vi "DAQ-Hybrid Engine-final.vi"() -> ()   [LabVIEW 2013]
uses:
  <vilib>/DAQmx/read.llb/DAQmx Read (Analog 1D Wfm NChan 1Samp).vi
  <vilib>/Analysis/baseanly.llb/Mean (DBL).vi
  <vilib>/DAQmx/read.llb/DAQmx Read (Analog Wfm 1Chan NSamp).vi
  <vilib>/DAQmx/read.llb/DAQmx Read (Analog Wfm 1Chan 1Samp).vi
  <vilib>/DAQmx/read.llb/DAQmx Read (Analog 1D DBL NChan 1Samp).vi
  <vilib>/DAQmx/configure/timing.llb/DAQmx Timing (Sample Clock).vi
  <vilib>/Utility/file.llb/Write To Spreadsheet File (string).vi
  <vilib>/Utility/file.llb/Write To Spreadsheet File (DBL).vi
  <vilib>/DAQmx/miscellaneous.llb/DAQmx Fill In Error Info.vi
  <vilib>/Analysis/NI_AALBase.lvlib
panel:
  in  "clear chart":bool
  out "?":dbl
  out "Servo":dbl(slide)=-430.10425378048984 scale=0.0..100.0
  out "?":dbl
  out "Chamber":dbl(slide)=-430.2760122999443 scale=0.0..100.0
  out "?":dbl
  out "Plumbing":dbl(slide)=-430.905793537944 scale=0.0..100.0
  out "?":dbl
  out "Pressure 2":dbl(knob) scale=0.0..2000.0
  in  "File Path 3":path=path "C:/Users/local-admin/Desktop/SRT-3 DAQ/test117.csv"
  out "?":dbl
  out "Ambient":dbl(slide)=-430.10425378048984 scale=0.0..100.0
  out "Waveform Chart":waveform(dbl)(graph)={"t0"=timestamp(3542319786.47639 s since 1904-01-01), "dt"=0.1, "Y"=[-147.1278504434858, -147.1152908145616], "attributes"=variant("NI_ChannelName"=variant(string "Voltage"), "NI_UnitDescription"=variant(string "Lbf"))}
  out "?":dbl
  out "Thrust":dbl(slide)=1.707317073170724 scale=-350.0..350.0
  out "?":dbl
  out "Plumbing":dbl(knob) scale=0.0..2000.0
  in  "?":bool
  in  "Samples Per Update":dbl=10.0
  in  "Sampling Rate [Hz]":i32=10
  # "Sampling Settings"
  # "Data Logging Settings"
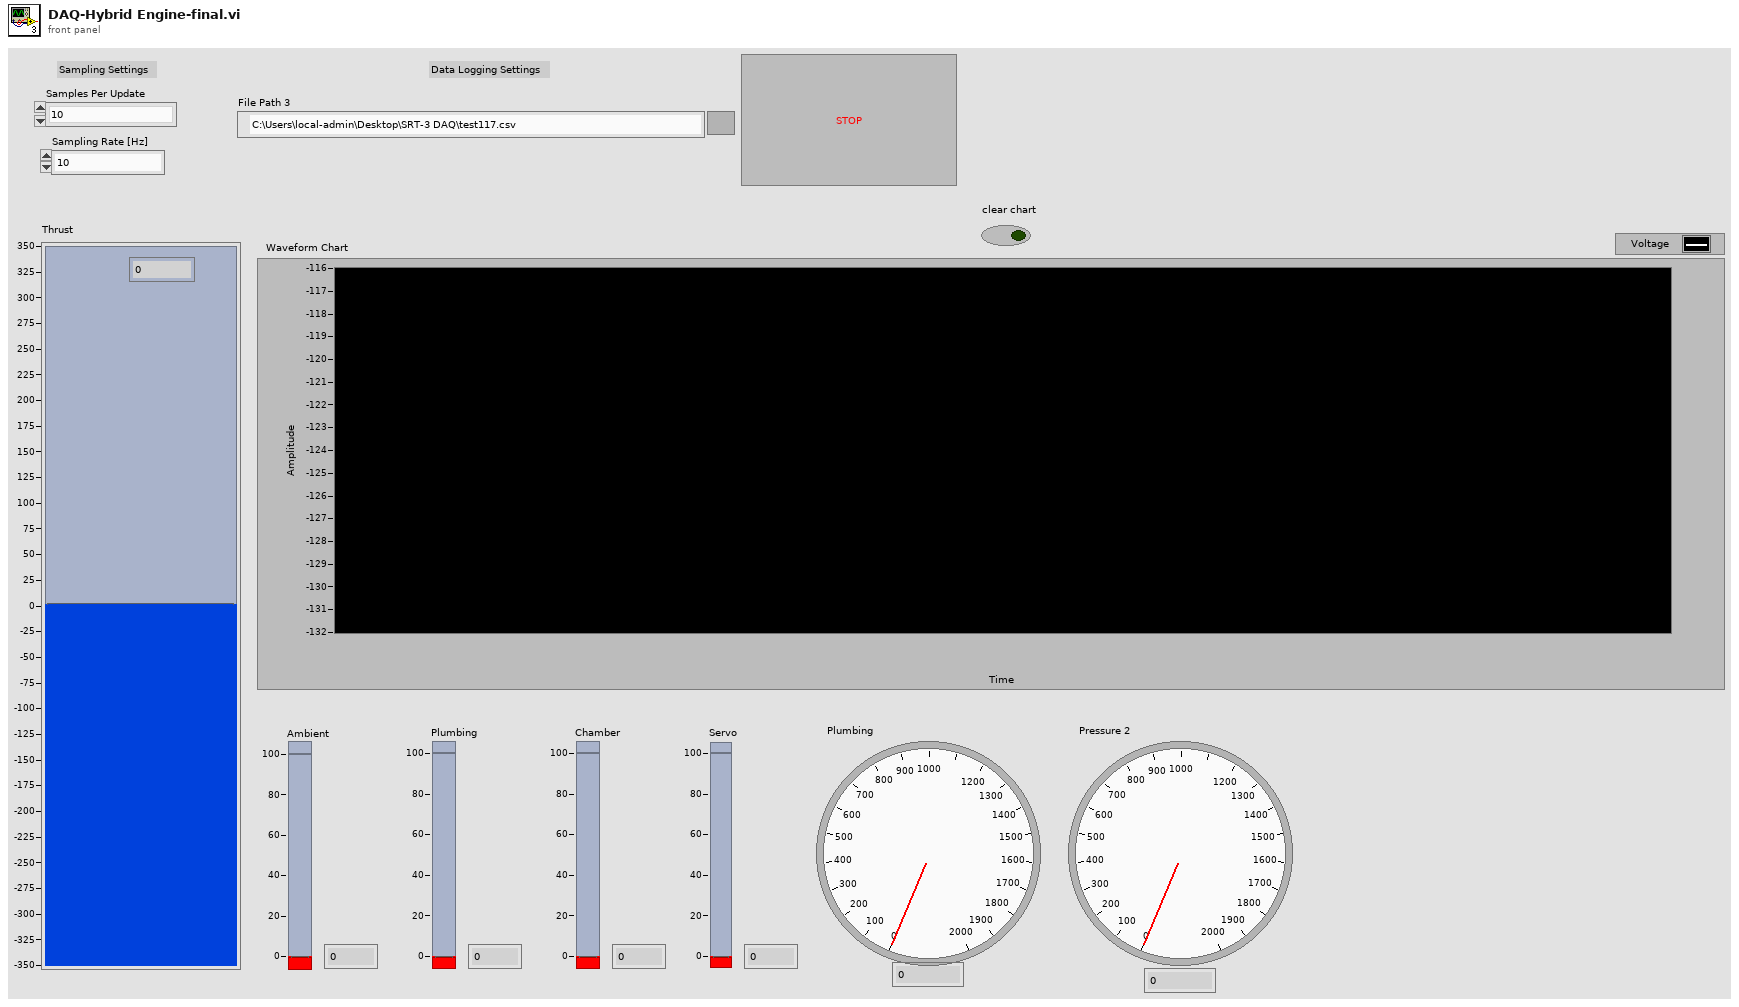
[diagram p1: front panel]
types:
  T1 = enum16{"open", "replace", "create", "open or create", "replace or create", "replace or create with confirmation"}
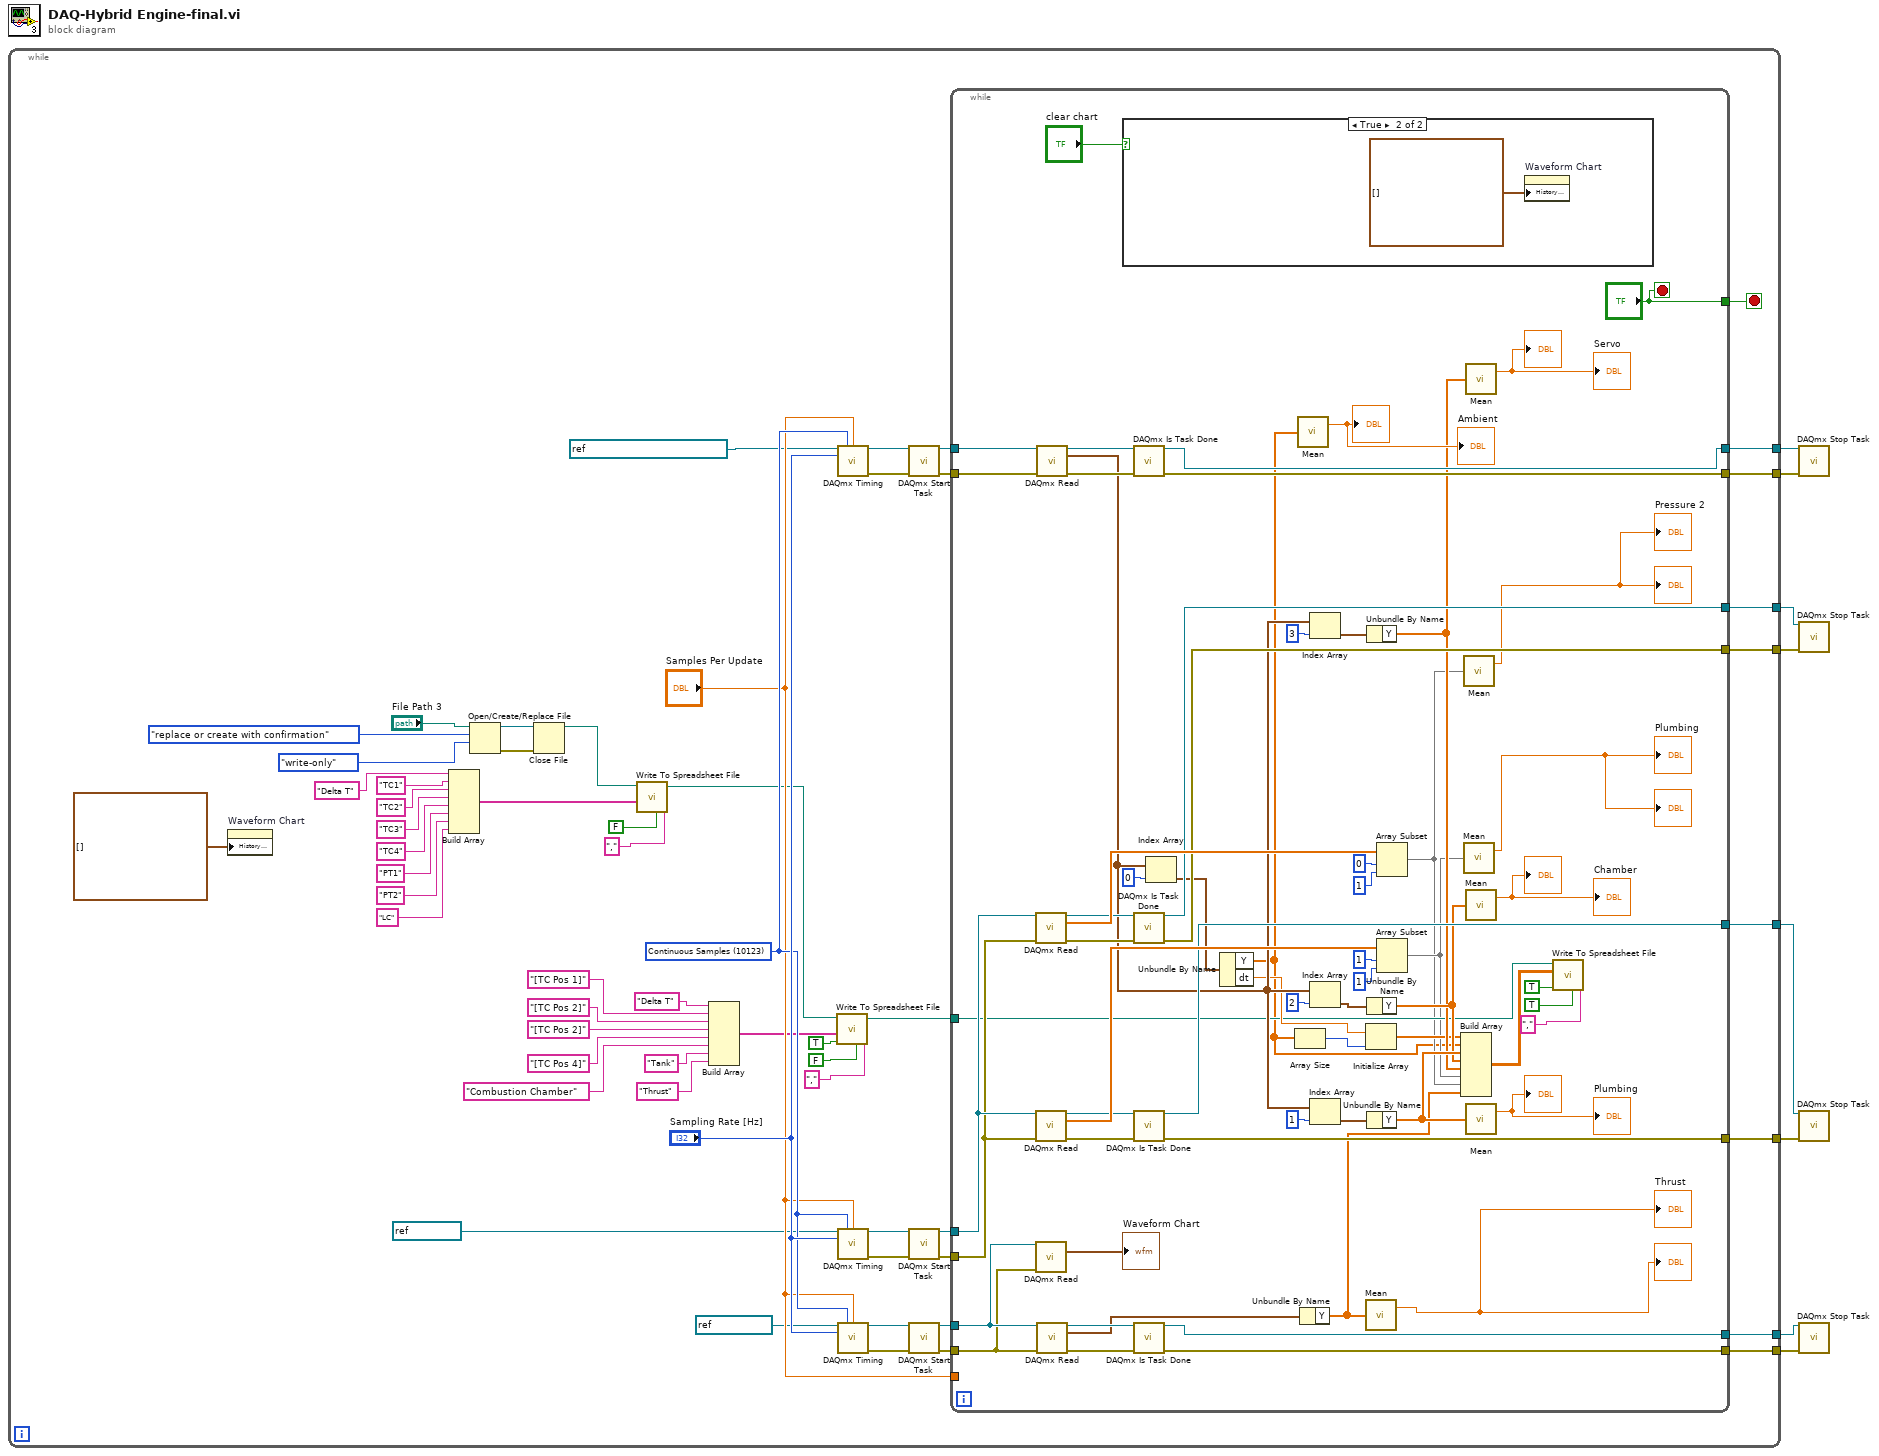
[diagram p0: block diagram]
diagram:
  n1 = while {
    tunnel: [w54] -> w8
    tunnel: [w53] -> w7
    tunnel: [w56] -> w6
    tunnel: [w55] -> w5
    tunnel: [w52] -> w4
    tunnel: [w51] -> w3
    tunnel: [w50] -> w2
    tunnel: [w49] -> w1
    stop <- w11 stop-if-true
    w61 = 10123 items=["Finite Samples"=10178, "Continuous Samples"=10123, "Hardware Timed Single Point"=12522] ("sample mode")
    n2 = property on="Waveform Chart" class="WFChart (strict)"("History Data"=waveform(dbl)[] []) -> ()  [unwired: 2 in, 2 out]
    n3 = Build Array("Delta T", "TC1", "TC2", "TC3", "TC4", "PT1", "PT2", "LC") -> (w31:string[])
    n4 = Open/Create/Replace File(file path (use dialog)="File Path 3", operation (0:open)=T1."replace or create with confirmation", access (0:read/write)=enum16{"read/write", "read-only", "write-only"}."write-only") -> (refnum out=w45:refnum<file>, error out=w44:errorcluster)  [unwired: 3 in, 1 out]
    n5 = Close File(refnum=w45, error in=w44) -> (path=w34:path)  [unwired: 1 out]
    n6 = call-poly <vilib>:"Write To Spreadsheet File.vi"("delimiter (\\t)"="," ("delimiter (\\t)"), "transpose? (no:F)"=FALSE, "1D data"=w31, "file path (dialog if empty)"=w34) -> ("new file path (Not A Path if cancelled)"=w20:path)  [unwired: 4 in]
    n7 = Build Array("Delta T", "[TC Pos 1]", "[TC Pos 2]", "[TC Pos 2]", "[TC Pos 4]", "Combustion Chamber", "Tank", "Thrust") -> (w16:string[])
    n8 = call-poly <vilib>:"Write To Spreadsheet File.vi"("delimiter (\\t)"="," ("delimiter (\\t)"), "transpose? (no:F)"=FALSE, "append to file? (new file:F)"=TRUE, "1D data"=w16, "file path (dialog if empty)"=w20) -> ("new file path (Not A Path if cancelled)"=w14:path)  [unwired: 3 in]
    n9 = call-poly <vilib>:"DAQmx Timing.vi"("task/channels in"=refnum<k21> "Thermocouple Channels" ("task in"), "sample mode"=w61, "samples per channel"="Samples Per Update", "rate"="Sampling Rate [Hz]") -> ("task out"=w59:refnum<k21>, "error out"=w58:errorcluster)  [unwired: 10 in]
    n10 = call-poly <vilib>:"DAQmx Timing.vi"("task/channels in"=refnum<k21> "PT 2000" ("task in"), "sample mode"=w61, "samples per channel"="Samples Per Update", "rate"="Sampling Rate [Hz]") -> ("task out"=w43:refnum<k21>, "error out"=w42:errorcluster)  [unwired: 10 in]
    n11 = call-poly <vilib>:"DAQmx Timing.vi"("task/channels in"=refnum<k21> "Load Cell" ("task in"), "sample mode"=w61, "samples per channel"="Samples Per Update", "rate"="Sampling Rate [Hz]") -> ("task out"=w41:refnum<k21>, "error out"=w40:errorcluster)  [unwired: 10 in]
    n12 = call <vilib>:"DAQmx Start Task.vi"("task/channels in"=w59, "error in"=w58) -> ("task out"=w63:refnum<k21>, "error out"=w57:errorcluster)  [unwired: 12 in]
    n13 = call <vilib>:"DAQmx Start Task.vi"("task/channels in"=w43, "error in"=w42) -> ("task out"=w67:refnum<k21>, "error out"=w66:errorcluster)  [unwired: 12 in]
    n14 = call <vilib>:"DAQmx Start Task.vi"("task/channels in"=w41, "error in"=w40) -> ("task out"=w65:refnum<k21>, "error out"=w64:errorcluster)  [unwired: 12 in]
    n15 = while {
      tunnel: w67 -> [w110]
      tunnel: w66 -> [w109]
      tunnel: ["?"] -> w11
      tunnel: w65 -> [w76]
      tunnel: w64 -> [w75]
      tunnel: "Samples Per Update" -> [_]
      tunnel: w63 -> [w101]
      tunnel: w57 -> [w127]
      tunnel: [w119] -> w56
      tunnel: [w118] -> w55
      tunnel: [w117] -> w54
      tunnel: [w116] -> w53
      tunnel: [w108] -> w52
      tunnel: [w107] -> w51
      tunnel: [w106] -> w50
      tunnel: [w105] -> w49
      tunnel: w14 -> [w81]
      stop <- "?" stop-if-true
      n16 = call-poly <vilib>:"DAQmx Read.vi"("task/channels in"=w110, "error in"=w109) -> ("task out"=w111:refnum<k21>, "data"=w114:dbl[], "error out"=w112:errorcluster)  [unwired: 11 in]
      n17 = call-poly <vilib>:"DAQmx Read.vi"("task/channels in"=w110, "error in"=w109) -> ("task out"=w124:refnum<k21>, "data"=w129:dbl[], "error out"=w125:errorcluster)  [unwired: 11 in]
      n18 = call-poly <vilib>:"DAQmx Read.vi"("task/channels in"=w76, "error in"=w75) -> ("data"=→"Waveform Chart":waveform(dbl))  [unwired: 11 in, 2 out]
      n19 = call-poly <vilib>:"DAQmx Read.vi"("task/channels in"=w101, "error in"=w127) -> ("task out"=w122:refnum<k21>, "data"=w97:waveform(dbl)[], "error out"=w123:errorcluster)  [unwired: 11 in]
      n20 = call-poly <vilib>:"DAQmx Read.vi"("task/channels in"=w76, "error in"=w75) -> ("task out"=w120:refnum<k21>, "data"=w74:waveform(dbl), "error out"=w121:errorcluster)  [unwired: 11 in]
      n21 = case shown="True" "clear chart" {
        frame False {
        }
        frame True {
          n22 = property on="Waveform Chart" class="WFChart (strict)"("History Data"=waveform(dbl)[] []) -> ()  [unwired: 2 in, 2 out]
        }
      }
      n23 = call <vilib>:"DAQmx Is Task Done.vi"("task/channels in"=w122, "error in"=w123) -> ("task out"=w106:refnum<k21>, "error out"=w105:errorcluster)  [unwired: 11 in, 1 out]
      n24 = call <vilib>:"DAQmx Is Task Done.vi"("task/channels in"=w111, "error in"=w112) -> ("task out"=w108:refnum<k21>, "error out"=w107:errorcluster)  [unwired: 11 in, 1 out]
      n25 = call <vilib>:"DAQmx Is Task Done.vi"("task/channels in"=w124, "error in"=w125) -> ("task out"=w117:refnum<k21>, "error out"=w116:errorcluster)  [unwired: 11 in, 1 out]
      n26 = call <vilib>:"DAQmx Is Task Done.vi"("task/channels in"=w120, "error in"=w121) -> ("task out"=w119:refnum<k21>, "error out"=w118:errorcluster)  [unwired: 11 in, 1 out]
      n27 = Index Array(array=w97, index=0) -> (element=w96:waveform(dbl))
      n28 = Unbundle By Name(w96) -> ("Y"=w78:dbl[], "dt"=w83:dbl)
      n29 = Array Size(array=w78) -> (size(s)=w84:i32)
      n30 = call-poly <vilib>:"Mean.vi"("X"=w78) -> ("mean"=→"Ambient" →"?":dbl)  [unwired: 1 out]
      n31 = Unbundle By Name(w74) -> ("Y"=w77:dbl[])
      n32 = Index Array(array=w97, index=3) -> (element=w93:waveform(dbl))
      n33 = Index Array(array=w97, index=2) -> (element=w94:waveform(dbl))
      n34 = Index Array(array=w97, index=1) -> (element=w95:waveform(dbl))
      n35 = Initialize Array(w83, w84) -> (w82:dbl[])
      n36 = call-poly <vilib>:"Mean.vi"("X"=w77) -> ("mean"=→"Thrust" →"?":dbl)  [unwired: 1 out]
      n37 = Unbundle By Name(w93) -> ("Y"=w86:dbl[])
      n38 = Unbundle By Name(w94) -> ("Y"=w87:dbl[])
      n39 = Unbundle By Name(w95) -> ("Y"=w88:dbl[])
      n40 = Array Subset(array=w114, index=0, length=1) -> (w79:dbl[])
      n41 = Array Subset(array=w129, index=1, length=1) -> (w80:dbl[])
      n42 = Build Array(w82, w78, w88, w87, w86, w80, w79, w77) -> (w85:dbl[][])
      n43 = call-poly <vilib>:"Mean.vi"("X"=w79) -> ("mean"=→"Pressure 2" →"?":dbl)  [unwired: 1 out]
      n44 = call-poly <vilib>:"Mean.vi"("X"=w80) -> ("mean"=→"Plumbing" →"?":dbl)  [unwired: 1 out]
      n45 = call-poly <vilib>:"Mean.vi"("X"=w86) -> ("mean"=→"Servo" →"?":dbl)  [unwired: 1 out]
      n46 = call-poly <vilib>:"Mean.vi"("X"=w87) -> ("mean"=→"Chamber" →"?":dbl)  [unwired: 1 out]
      n47 = call-poly <vilib>:"Mean.vi"("X"=w88) -> ("mean"=→"Plumbing" →"?":dbl)  [unwired: 1 out]
      n48 = call-poly <vilib>:"Write To Spreadsheet File.vi"("delimiter (\\t)"="," ("delimiter (\\t)"), "transpose? (no:F)"=TRUE, "append to file? (new file:F)"=TRUE, "2D data"=w85, "file path (dialog if empty)"=w81) -> ()  [unwired: 3 in, 1 out]
    }
  }
  n49 = call <vilib>:"DAQmx Stop Task.vi"("task/channels in"=w2, "error in"=w1) -> ()  [unwired: 12 in, 2 out]
  n50 = call <vilib>:"DAQmx Stop Task.vi"("task/channels in"=w4, "error in"=w3) -> ()  [unwired: 12 in, 2 out]
  n51 = call <vilib>:"DAQmx Stop Task.vi"("task/channels in"=w8, "error in"=w7) -> ()  [unwired: 12 in, 2 out]
  n52 = call <vilib>:"DAQmx Stop Task.vi"("task/channels in"=w6, "error in"=w5) -> ()  [unwired: 12 in, 2 out]
